vi "intDivide.vi"() -> ()   [LabVIEW 2011, in "IntClass.lvclass"]
uses:
  IntClass.lvclass
panel:
  out "floor(Int1/Int2)":refnum<class "IntClass.lvclass">
  in  "Int2 in":refnum<class "IntClass.lvclass">
  out "Timing":u32
  out "Error out":errorcluster
  in  "Error in (no error)":errorcluster
  out "Int1 - Int2*floor(Int1/Int2)":refnum<class "IntClass.lvclass">
  in  "Int1 in":refnum<class "IntClass.lvclass">
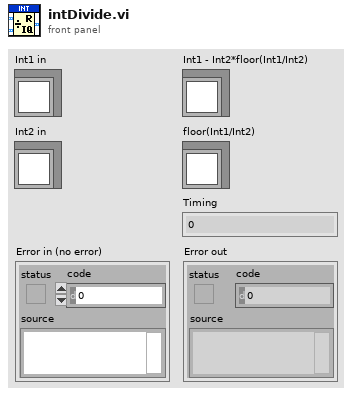
[diagram p1: front panel]
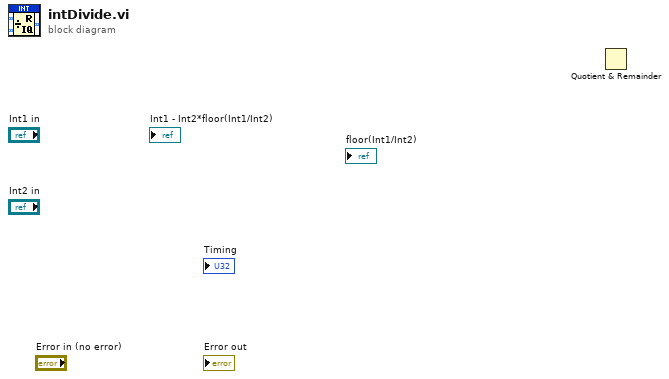
[diagram p0: block diagram]
diagram:
  n1 = Quotient & Remainder() -> ()  [unwired: 2 in, 2 out]
